vi "Update Table Buffer Pressure.vi"(7 "BUFFER Ref":refnum<vi>, 8 "error in (no error)":errorcluster, 11 "Table Buffer Pressure Ref":refnum<vi>) -> (0 "error out":errorcluster)   [LabVIEW 2025, in "I2C Bus Monitor UI.lvlib"]
uses:
  I2C Bus Monitor UI.lvlib
  Table Buffer - Check.vi
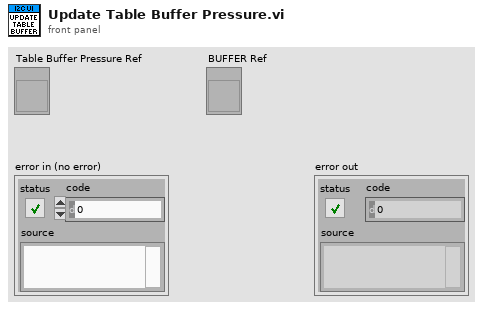
[diagram p1: front panel]
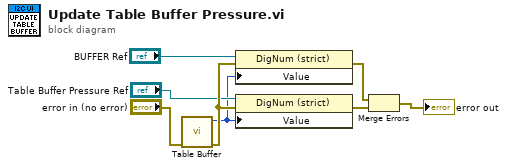
[diagram p0: block diagram]
diagram:
  n1 = call-poly "Table Buffer.vi"("error in (no error)"="error in (no error)") -> ("error out"=w8:errorcluster, "# elements in queue"=w3:i32)  [unwired: 9 in]
  n2 = property class="DigNum (strict)"(reference="BUFFER Ref", error in=w8, "Value"=w3) -> (error out=w1:errorcluster)  [unwired: 1 out]
  n3 = property class="DigNum (strict)"(reference="Table Buffer Pressure Ref", error in=w8, "Value"=w3) -> (error out=w6:errorcluster)  [unwired: 1 out]
  n4 = Merge Errors(w1, w6) -> (→"error out":errorcluster)
